vi "gen MB frame_ turn the relay ON_OFF.vi"(9 "ON OFF":bool, 10 "Relay IDs":u16, 11 "Dev addr":u8=1 format="%x") -> (3 "MB frame":string)   [LabVIEW 2016, in "MB _relays.lvlib"]
uses:
  MB _relays.lvlib
  type defs/Relay State.ctl
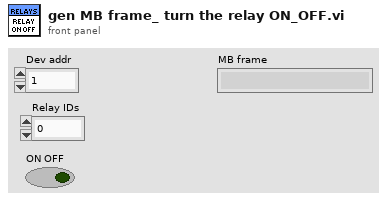
[diagram p1: front panel]
types:
  T1 = typedef "MB _relays.lvlib/Relay State.ctl" = u16
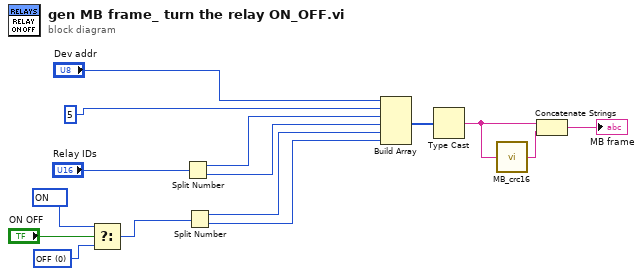
[diagram p0: block diagram]
diagram:
  w2 = T1 0 items=["ON"=65280, "OFF"=0] ("ON_OFF")
  w4 = T1 65280 items=["ON"=65280, "OFF"=0] ("ON_OFF")
  n1 = Select(t=w4, s="ON OFF", f=w2) -> (s? t:f=w1:T1)
  n2 = Split Number(x="Relay IDs") -> (hi(x)=w14:u8, lo(x)=w13:u8)
  n3 = Split Number(x=w1) -> (hi(x)=w12:u8, lo(x)=w11:u8)
  n4 = Build Array("Dev addr", u8 5, w14, w13, w12, w11) -> (w10:u8[])
  n5 = Type Cast(x=w10) -> (*(type *) &x=w7:string)  [unwired: 1 in]
  n6 = call "MB_crc16.vi"("message"=w7) -> ("CRC16"=w8:string)  [unwired: 4 in]
  n7 = Concatenate Strings(w7, w8) -> (→"MB frame":string)
